vi "String - Extract _Body_.vi"(10 "Temp Array":string[](array[string]), 11 "<wps>":T1) -> (3 "<rev>":string[](array[string]))   [LabVIEW 2013]
uses:
  Controls/Combo Box.ctl
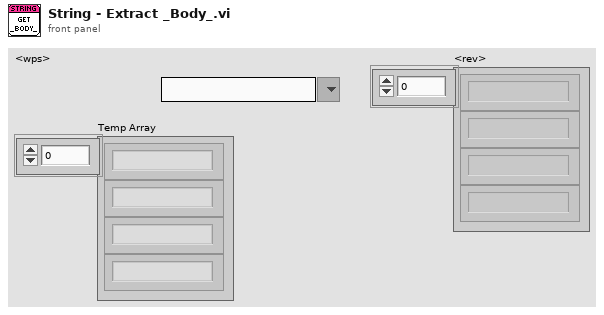
[diagram p1: front panel]
types:
  T1 = typedef "Combo Box.ctl" = string
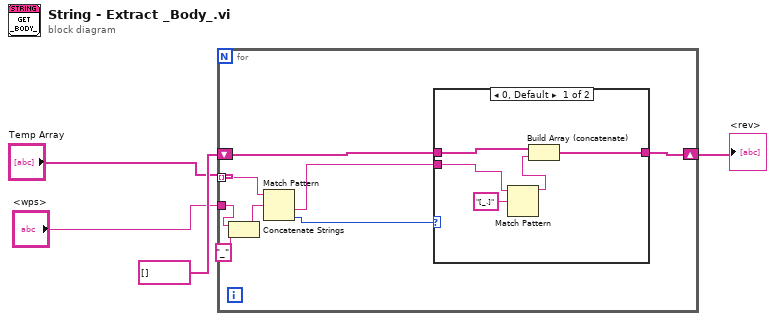
[diagram p0: block diagram]
diagram:
  n1 = for {
    tunnel: "Temp Array" -> [w12] mode=indexing
    tunnel: "<wps>" -> [w10]
    shift-right: [w6] -> w4
    shift-left: string[] [] -> [w5]
    n2 = Concatenate Strings(w10, "_" ("string")) -> (w8:string)
    n3 = Match Pattern(string=w12, regular expression=w8) -> (after substring=w7:string, offset past match=w11:i32)  [unwired: 1 in, 2 out]
    n4 = case shown="0, Default" w11 {
      tunnel: w7 -> [w15 _]
      tunnel: [w17 w18] -> w6
      tunnel: w5 -> [w16 w18]
      frame 0, Default {
        n5 = Match Pattern(string=w15, regular expression="[_.]") -> (before substring=w13:string)  [unwired: 1 in, 3 out]
        n6 = Build Array (concatenate)(w16, w13) -> (w17:string[])
      }
      frame -1 {
      }
    }
  }
  "<rev>" <- w4
